vi "Main Simon Says.vi"() -> ()   [LabVIEW 2017]
uses:
  Controls/Sequence.ctl
  Controls/Events.ctl
panel:
  out "Level":i32
  in  "Sequence":T1
  in  "Stop":bool
  in  "Start":bool
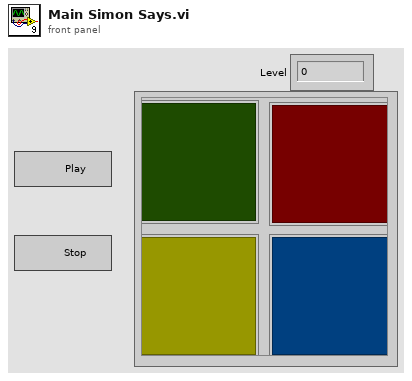
[diagram p1: front panel]
types:
  T1 = typedef "Sequence.ctl" = cluster{"S1":bool, "S2":bool, "S3":bool, "S4":bool}
  T2 = typedef "Events.ctl" = enum16{"Inicializar", "Event Handler", "New Sequence", "Compare Sequence", "Stop"}
  T3 = enum8{"Enabled", "Disabled", "Disabled and Grayed Out"}
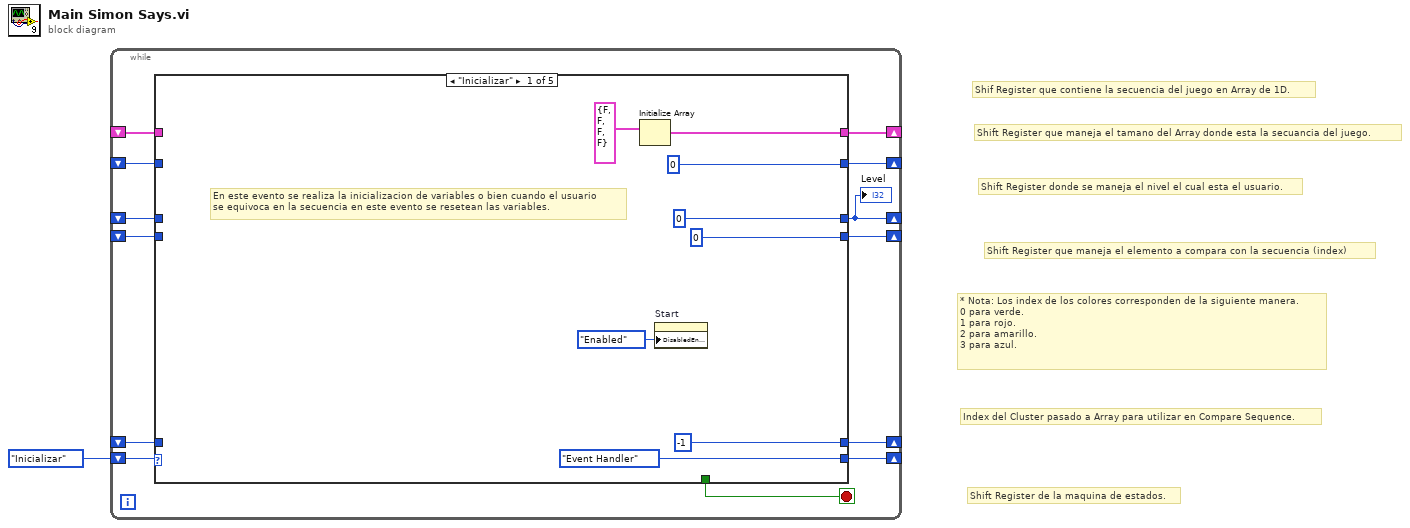
[diagram p0: block diagram]
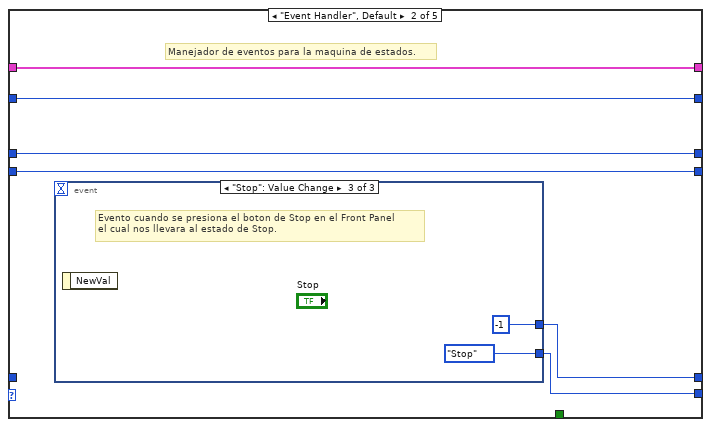
[diagram p2: hidden frame]
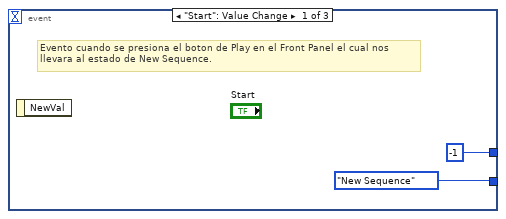
[diagram p3: hidden frame]
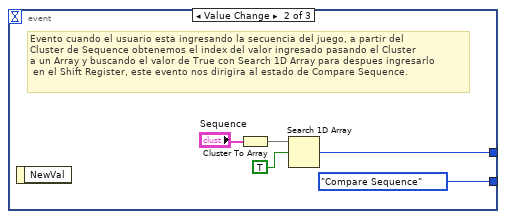
[diagram p4: hidden frame]
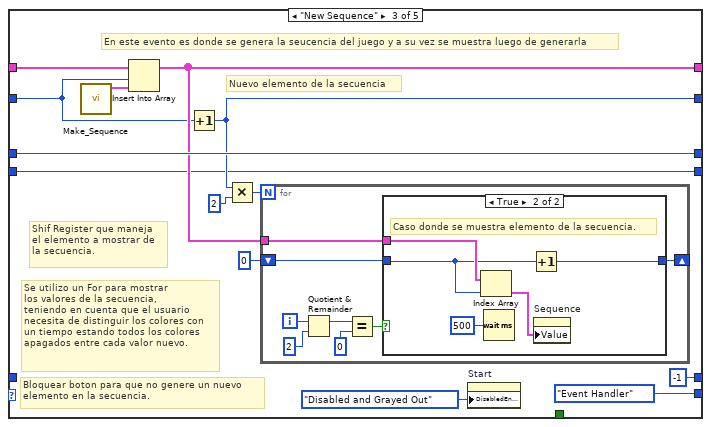
[diagram p5: hidden frame]
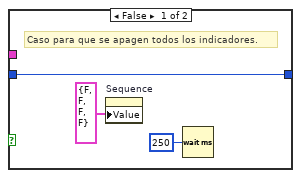
[diagram p6: hidden frame]
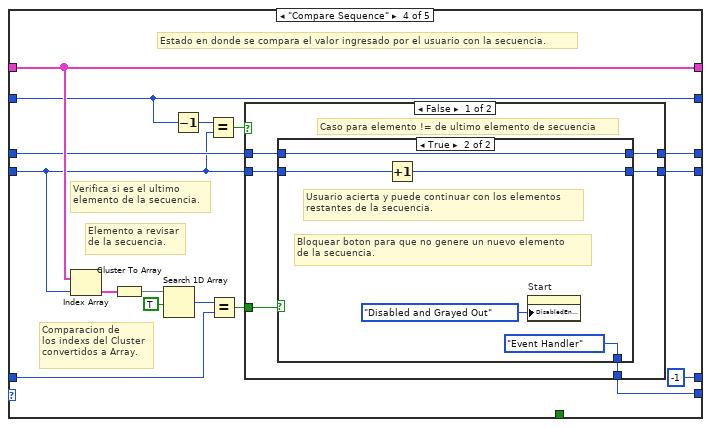
[diagram p7: hidden frame]
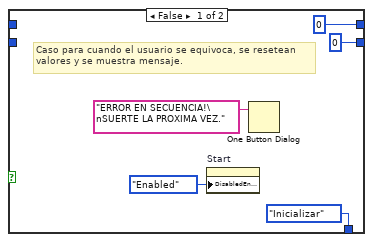
[diagram p8: hidden frame]
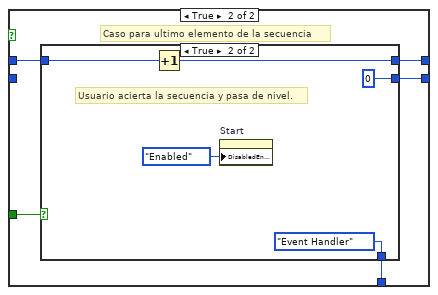
[diagram p9: hidden frame]
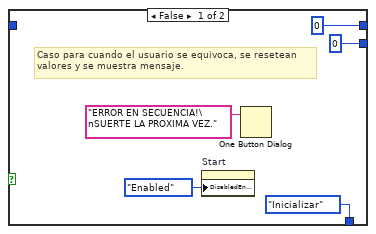
[diagram p10: hidden frame]
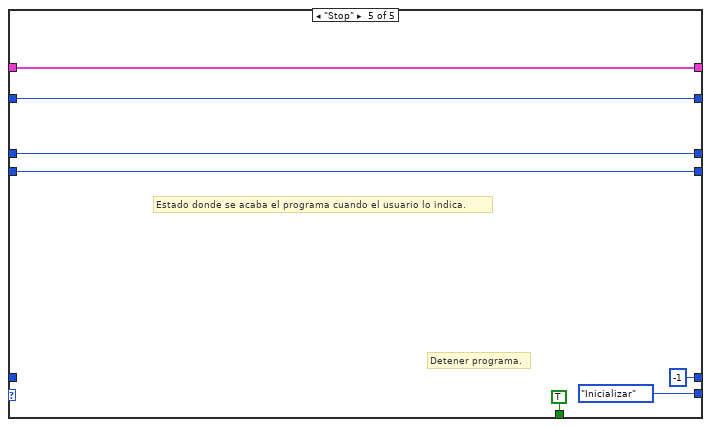
[diagram p11: hidden frame]
diagram:
  # "* Nota: Los index de los colores corresponden de la siguiente manera.\n0 para verde.\n1 para rojo.\n2 para amarillo.\n3 para azul."
  # "Index del Cluster pasado a Array para utilizar en Compare Sequence."
  # "Shift Register de la maquina de estados."
  # "Shift Register que maneja el elemento a compara con la secuencia (index)"
  # "Shift Register donde se maneja el nivel el cual esta el usuario."
  # "Shift Register que maneja el tamano del Array donde esta la secuancia del juego."
  # "Shif Register que contiene la secuencia del juego en Array de 1D."
  n1 = while {
    shift-right: [w12] -> _
    shift-left: _ -> [w11]
    shift-right: [w13] -> _
    shift-left: _ -> [w8]
    shift-right: [w10] -> _
    shift-left: _ -> [w9]
    shift-right: [w6] -> _
    shift-left: Events."Inicializar" -> [w14]
    shift-right: [w5] -> _
    shift-left: _ -> [w4]
    shift-right: [w3] -> _
    shift-left: _ -> [w2]
    stop <- w7 stop-if-true
    n2 = case shown="\"Inicializar\"" w14 {
      tunnel: [0 w28 w48 w73 w118] -> w13
      tunnel: [w21 w26 w47 w81 w120] -> w12
      tunnel: w11 -> [_ w26 w50 w81 w120]
      tunnel: [0 ("index") w27 w43 w70 w119] -> w10
      tunnel: w9 -> [_ w27 w46 w70 w119]
      tunnel: w8 -> [_ w28 w48 w71 w118]
      tunnel: [_ _ _ _ TRUE] -> w7
      tunnel: [Events."Event Handler" w25 Events."Event Handler" w68 Events."Inicializar"] -> w6
      tunnel: [-1 ("index of element") w24 -1 ("index of element") -1 ("index of element") -1 ("index of element")] -> w5
      tunnel: w4 -> [_ _ _ w76 _]
      tunnel: [0 ("index") w23 w39 w72 w114] -> w3
      tunnel: w2 -> [_ w23 w39 w67 w114]
      frame "Inicializar" {
        # "En este evento se realiza la inicializacion de variables o bien cuando el usuario \nse equivoca en la secuencia en este evento se resetean las variables."
        n3 = Initialize Array(T1 {"S1"=FALSE, "S2"=FALSE, "S3"=FALSE, "S4"=FALSE} ("Sequence")) -> (w21:T1[])  [unwired: 1 in]
        n4 = property on="Start" class="Bool"("DisabledEnum"=T3."Enabled" ("Disabled")) -> ()  [unwired: 2 in, 2 out]
      }
      frame "Event Handler", Default {
        # "Manejador de eventos para la maquina de estados."
        n5 = event shown="[2] \"Stop\": Value Change" {
          selector: _ -> [_ _ _]
          dyn-events: _ -> [_ _ _]
          timeout: _ -> [_ _ _]
          tunnel: [Events."New Sequence" Events."Compare Sequence" Events."Stop"] -> w25
          tunnel: [-1 ("index of element") w32 -1 ("index of element")] -> w24
          event "Start": Value Change {
            # "Evento cuando se presiona el boton de Play en el Front Panel el cual nos\nllevara al estado de New Sequence."
            n6 = event-data() -> ()  [unwired: 1 in, 1 out]
          }
          event Value Change {
            # "Evento cuando el usuario esta ingresando la secuencia del juego, a partir del \nCluster de Sequence obtenemos el index del valor ingresado pasando el Cluster\na un Array y buscando el valor de True con Search 1D Array para despues ingresarlo\n en el Shift Register, este evento nos dirigira al estado de Compare Sequence."
            n7 = event-data() -> ()  [unwired: 1 in, 1 out]
            n8 = Cluster To Array(cluster="Sequence") -> (array=w34:bool[])
            n9 = Search 1D Array(1D array=w34, element=TRUE) -> (index of element=w32:i32)  [unwired: 1 in]
          }
          event "Stop": Value Change {
            # "Evento cuando se presiona el boton de Stop en el Front Panel \nel cual nos llevara al estado de Stop."
            n10 = event-data() -> ()  [unwired: 1 in, 1 out]
          }
        }
      }
      frame "New Sequence" {
        # "Bloquear boton para que no genere un nuevo\nelemento en la secuencia."
        # "Shif Register que maneja\nel elemento a mostrar de \nla secuencia."
        # "Se utilizo un For para mostrar\nlos valores de la secuencia,\nteniendo en cuenta que el usuario\nnecesita de distinguir los colores con\nun tiempo estando todos los colores\napagados entre cada valor nuevo."
        # "Nuevo elemento de la secuencia"
        # "En este evento es donde se genera la seucencia del juego y a su vez se muestra luego de generarla"
        n11 = call "Make_Sequence.vi"() -> ("Sequence"=w49:T1)  [unwired: 11 in]
        n12 = Insert Into Array(array=w50, index=w46, new element=w49) -> (w47:T1[])
        n13 = Increment(x=w46) -> (x+1=w43:i32)
        n14 = Multiply(x=w43, y=2) -> (x*y=w44:i32)
        n15 = for {
          N: w44 -> [_]
          tunnel: w47 -> [w51]
          shift-right: [w52] -> _
          shift-left: 0 ("y") -> [w53]
          i -> [w58]
          n16 = Quotient & Remainder(x=w58, y=2) -> (x-y*floor(x/y)=w56:i32)  [unwired: 1 out]
          n17 = Equal?(x=w56, y=0) -> (x = y?=w54:bool)
          n18 = case shown="True" w54 {
            tunnel: w53 -> [w60 w62]
            tunnel: [w60 w63] -> w52
            tunnel: w51 -> [_ w66]
            frame False {
              # "Caso para que se apagen todos los indicadores."
              n19 = property on="Sequence" class="Clust"("Value"=T1 {"S1"=FALSE, "S2"=FALSE, "S3"=FALSE, "S4"=FALSE} ("Sequence")) -> ()  [unwired: 2 in, 2 out]
              n20 = Wait (ms)(milliseconds to wait=u32 250) -> ()  [unwired: 1 out]
            }
            frame True {
              # "Caso donde se muestra elemento de la secuencia."
              n21 = Index Array(array=w66, index=w62) -> (element=w65:T1)
              n22 = Wait (ms)(milliseconds to wait=u32 500) -> ()  [unwired: 1 out]
              n23 = Increment(x=w62) -> (x+1=w63:i32)
              n24 = property on="Sequence" class="Clust"("Value"=w65) -> ()  [unwired: 2 in, 2 out]
            }
          }
        }
        n25 = property on="Start" class="Bool"("DisabledEnum"=T3."Disabled and Grayed Out" ("Disabled")) -> ()  [unwired: 2 in, 2 out]
      }
      frame "Compare Sequence" {
        # "Verifica si es el ultimo\nelemento de la secuencia."
        # "Comparacion de \nlos indexs del Cluster\nconvertidos a Array."
        # "Elemento a revisar\nde la secuencia."
        # "Estado en donde se compara el valor ingresado por el usuario con la secuencia."
        n26 = Index Array(array=w81, index=w67) -> (element=w80:T1)
        n27 = Cluster To Array(cluster=w80) -> (array=w79:bool[])
        n28 = Search 1D Array(1D array=w79, element=TRUE) -> (index of element=w77:i32)  [unwired: 1 in]
        n29 = Decrement(x=w70) -> (x-1=w69:i32)
        n30 = Equal?(x=w69, y=w67) -> (x = y?=w75:bool)
        n31 = Equal?(x=w77, y=w76) -> (x = y?=w74:bool)
        n32 = case shown="False" w75 {
          tunnel: w71 -> [w88 w103]
          tunnel: w74 -> [w87 w102]
          tunnel: [w86 w101] -> w73
          tunnel: [w85 w100] -> w72
          tunnel: w67 -> [w84 _]
          tunnel: [w83 w99] -> w68
          frame False {
            # "Caso para elemento != de ultimo elemento de secuencia"
            n33 = case shown="True" w87 {
              tunnel: w88 -> [_ w94]
              tunnel: [0 w94] -> w86
              tunnel: [0 w98] -> w85
              tunnel: w84 -> [_ w97]
              tunnel: [Events."Inicializar" Events."Event Handler"] -> w83
              frame False {
                # "Caso para cuando el usuario se equivoca, se resetean\nvalores y se muestra mensaje."
                n34 = property on="Start" class="Bool"("DisabledEnum"=T3."Enabled" ("Disabled")) -> ()  [unwired: 2 in, 2 out]
                n35 = One Button Dialog(message="ERROR EN SECUENCIA!\nSUERTE LA PROXIMA VEZ.") -> ()  [unwired: 1 in, 1 out]
              }
              frame True {
                # "Bloquear boton para que no genere un nuevo elemento\nde la secuencia."
                # "Usuario acierta y puede continuar con los elementos\nrestantes de la secuencia."
                n36 = Increment(x=w97) -> (x+1=w98:i32)
                n37 = property on="Start" class="Bool"("DisabledEnum"=T3."Disabled and Grayed Out" ("Disabled")) -> ()  [unwired: 2 in, 2 out]
              }
            }
          }
          frame True {
            # "Caso para ultimo elemento de la secuencia"
            n38 = case shown="True" w102 {
              tunnel: w103 -> [_ w111]
              tunnel: [0 w112] -> w101
              tunnel: [0 0] -> w100
              tunnel: [Events."Inicializar" Events."Event Handler"] -> w99
              frame False {
                # "Caso para cuando el usuario se equivoca, se resetean\nvalores y se muestra mensaje."
                n39 = property on="Start" class="Bool"("DisabledEnum"=T3."Enabled" ("Disabled")) -> ()  [unwired: 2 in, 2 out]
                n40 = One Button Dialog(message="ERROR EN SECUENCIA!\nSUERTE LA PROXIMA VEZ.") -> ()  [unwired: 1 in, 1 out]
              }
              frame True {
                # "Usuario acierta la secuencia y pasa de nivel."
                n41 = Increment(x=w111) -> (x+1=w112:i32)
                n42 = property on="Start" class="Bool"("DisabledEnum"=T3."Enabled" ("Disabled")) -> ()  [unwired: 2 in, 2 out]
              }
            }
          }
        }
      }
      frame "Stop" {
        # "Detener programa."
        # "Estado donde se acaba el programa cuando el usuario lo indica."
      }
    }
    "Level" <- w13
  }
